vi "CPP-BLplotter.vi"(1 "Job Directory":path) -> (2 "Saved Automatically?":bool, 3 "gnuplotScript":string, 4 "Plot data file":path)   [LabVIEW 2021]
uses:
  gnuplotScriptComponents/BLPlottersubVIs/BLTarget.ctl
  gnuplotScriptComponents/BLPlottersubVIs/Resampler.ctl
  gnuplotScriptComponents/at.ctl
  Results_plotter_Global.vi
  Data plotting/subVIs/Plot_Values_Global.vi
panel:
  in  "Tab Control":enum32{"Good Shit", "Targets", "Boring Shit"}(tab)
  in  "chooseSpectra":bool
  in  "Ref":enum32{"MS", "FS"}(radio)
  in  "Zref":dbl=508.0 min=0.0 step=25.0
  in  "h":dbl[unit] min=0.0 step=0.0005
  in  "NormaliseHeight?":bool
  in  "oneshot":bool=TRUE
  in  "U(h)":dbl[unit] min=0.0 step=0.5
  in  "Fit Zmin(mm)":dbl=100.0 min=0.0 max=200.0 step=20.0
  in  "autoprint":bool
  out "Power fit with d0":cluster{"n":dbl, "d0":dbl, "d0 2":dbl} {"d0 2" format="%#.1e"; "d0" format="%#.1f"; "n" format="%.3f"}
  in  "Fit Zmax(mm)":dbl=550.0 min=0.0 max=2000.0 step=50.0
  out "lambda-":dbl format="%_2g"
  out "lambda+":dbl format="%_2g"
  out "lambda(h)":dbl format="%.3g"
  in  "HeightJitter%":dbl min=0.0 max=20.0 step=1.0
  out "Spectrum":cluster{"all rows":dbl[], "all rows":dbl[]}[](graph)
  in  "Stop Button":bool
  in  "Print Button":bool
  out "U,L(U)":cluster{"Array":dbl[], "Array":dbl[]}[](graph)
  out "TI,Sigma":cluster{"Array":dbl[], "Array":dbl[]}[](graph)
  in  "MaxFitFreq":dbl=500.0
  in  "lambdaSpan(%)":dbl=20.0
  out "case":string
  out "Power fit No d0":cluster{"n":dbl, "d0":dbl, "d0 2":dbl} {"d0 2" format="%#.1e"; "n" format="%.3f"}
  in  "Spectra?":bool
  in  "Scale":u16=350 min=1 max=10000 step=50
  in  "Load BL Targets":bool
  in  "BL Scratchpad":T1[](array[typedef]) {"n" min=0.02 max=0.5 step=0.01 format="%.2f"}
  out "BL Targets":T1[](array[typedef]) {"n" min=0.02 max=0.5 step=0.01 format="%.2f"}
  out "FileName":string
  in  "Values to include in Page Title":i32[](listbox)
  out "ZrefMSmm":dbl
  in  "Units":enum16{"Metric", "English"}(ring)
  out "filenameNotes":string
  in  "ScaleInTitle?":bool
  in  "OutputType":enum16{"PDF", "PNG-ReportStyle"}(ring)
  out "outputPath":path
  in  "Resampler":T2
  in  "ResampleToN":i32=12
  in  "ResampleHeights":dbl[](array[numeric])=[25.4, 38.1, 50.8, 76.2, 101.6, 127.0, 152.4, 203.2, 254.0, 304.8, 406.4, 508.0, 609.6, 812.8, 1219.2, 1524.0]
  in  "Use for:":T3(array[ring])=[enum."\nU", enum."\nTI", enum."\nLambda", enum."\nSigma"]
  out "Incoming Titles":string[](array[string])
  out "Final Title":string
  in  "Plot Title Post Block":string
  in  "Plot Title Pre Block":string="Test"
  in  "Show Script Editor?":bool
  in  "OpenLogfile?":bool
  out "spectraLegend":string[](array[string])
  in  "SpecificPlotFolder":string="EnterSpecificPlotFolder"
  # "Fit using values at  measurement Z heights"
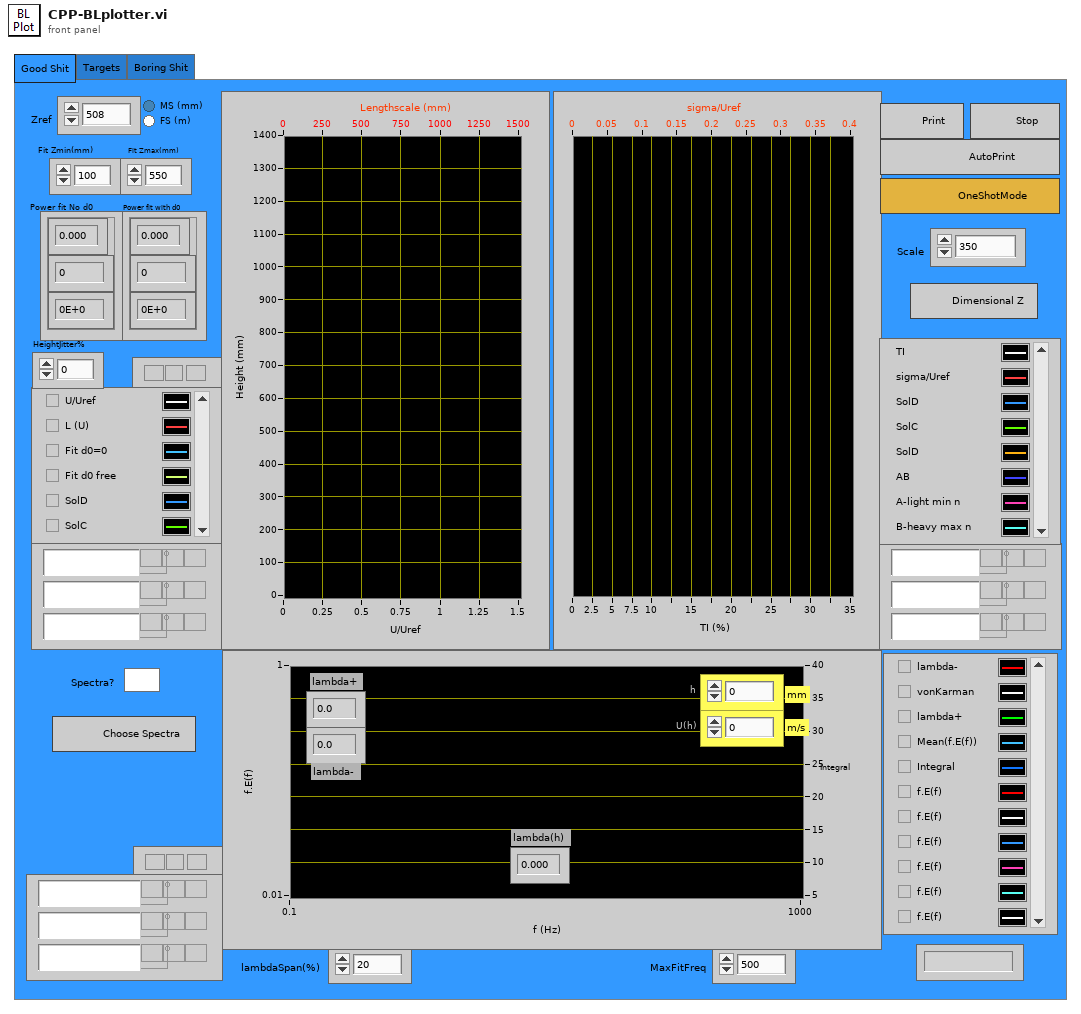
[diagram p1: front panel]
types:
  T1 = typedef "BLTarget.ctl" = cluster{"Code":string, "n":dbl, "Z:FS:(m)":dbl[], "U:FS:(m/s)":dbl[], "TI::(%)":dbl[]}
  T2 = typedef "Resampler.ctl" = enum32{"AsTaken", "Regular", "Prescribed"}
  T3 = enum16{"Don't Use", "\nU", "\nLambda", "\nTI", "\nSigma"}[]
  T4 = typedef "Error_bars.ctl" = cluster{"Upper":string[], "Lower":string[], "St Error":string[]}
  T5 = typedef "at.ctl" = cluster{"XcoordSys":string, "YcoordSys":string, "Xvalue":dbl, "Yvalue":dbl}
  T6 = typedef "LVRangeTypeDef.ctl" = cluster{"Minimum":dbl, "Maximum":dbl, "Increment":dbl, "Minor Increment":dbl, "Start":dbl}
  T7 = typedef "PowerLaw.ctl" = cluster{"n":dbl, "d0":dbl, "Residual":dbl}
  T8 = cluster{"Array":dbl[], "best nonlinear fit":dbl[]}
  T9 = cluster{"Plot.Plot Name":string, "Plot.Plot Color":u32, "Plot.Visible?":bool}
  T10 = typedef "minAndMax.ctl" = cluster{"Min":T11, "Max":T11}
  T11 = typedef "AutoManualNumber.ctl" = cluster{"Auto":bool, "Value":dbl}
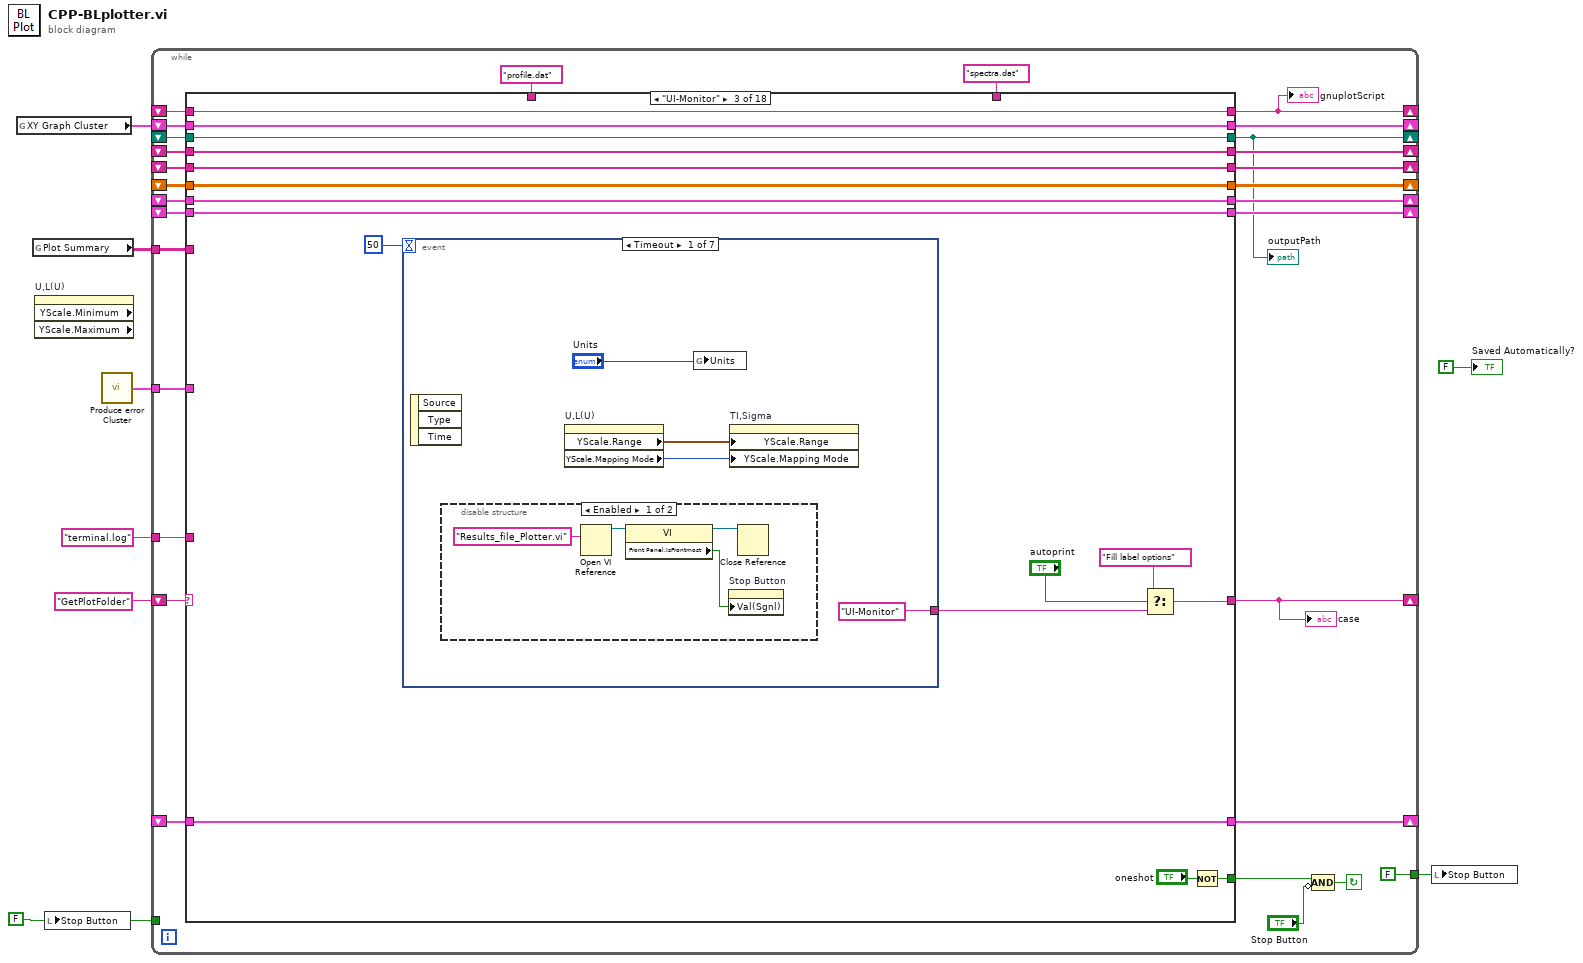
[diagram p0: block diagram]
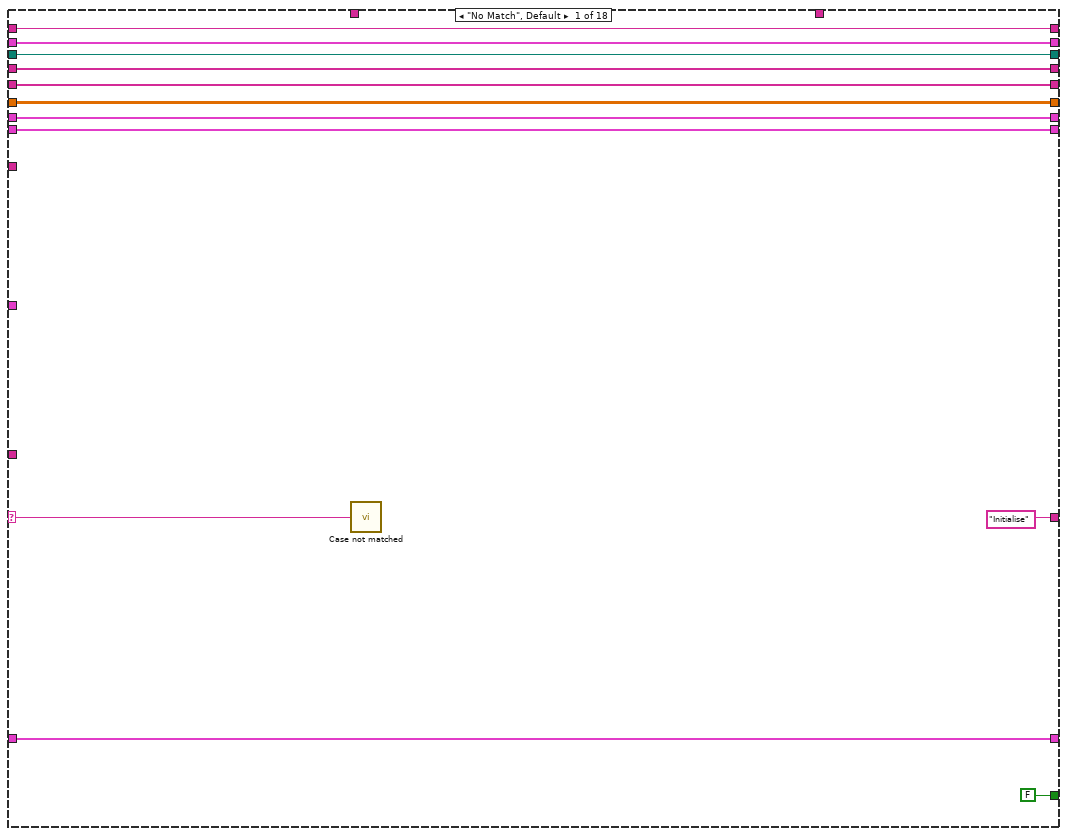
[diagram p2: hidden frame]
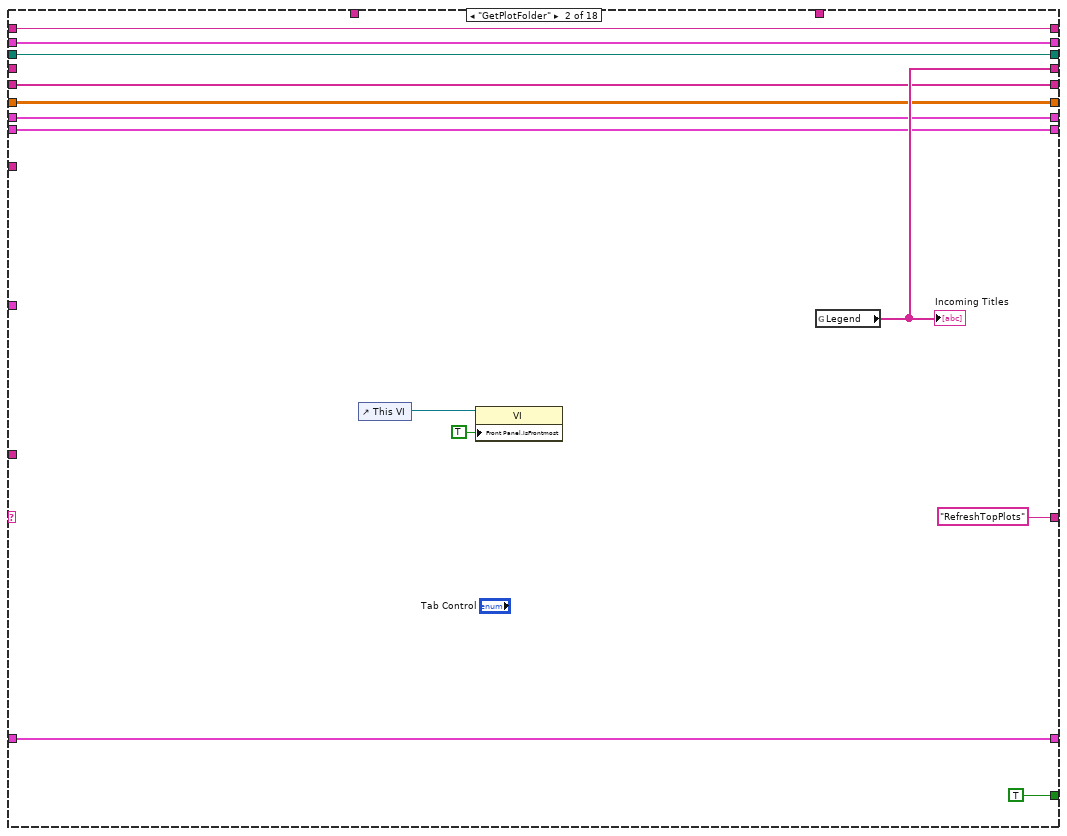
[diagram p3: hidden frame]
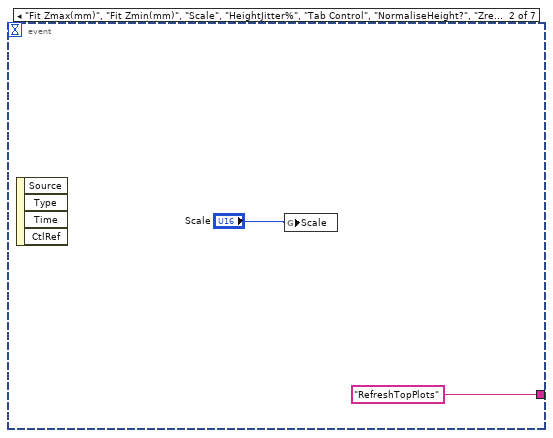
[diagram p5: hidden frame]
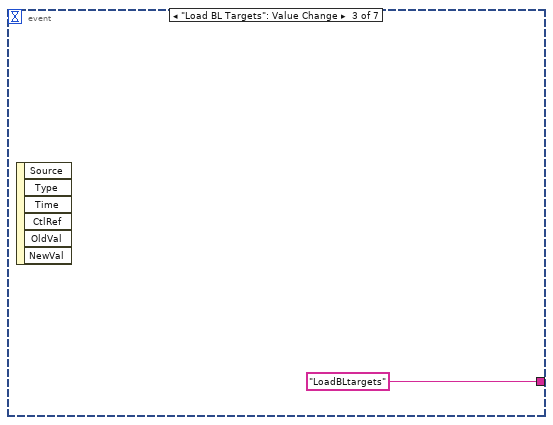
[diagram p6: hidden frame]
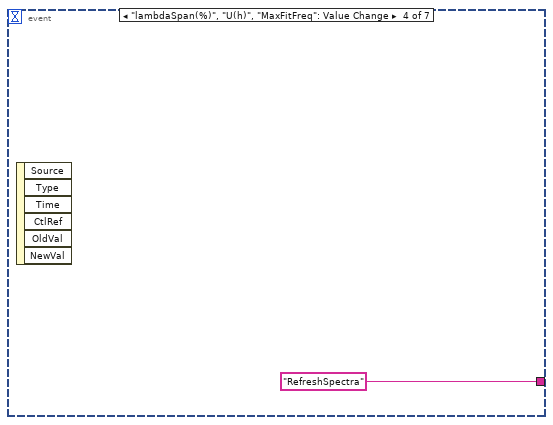
[diagram p7: hidden frame]
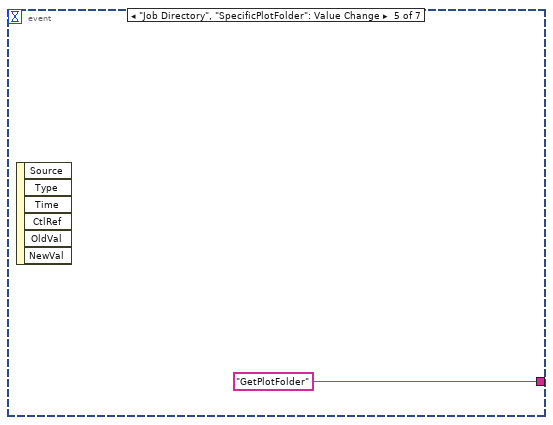
[diagram p8: hidden frame]
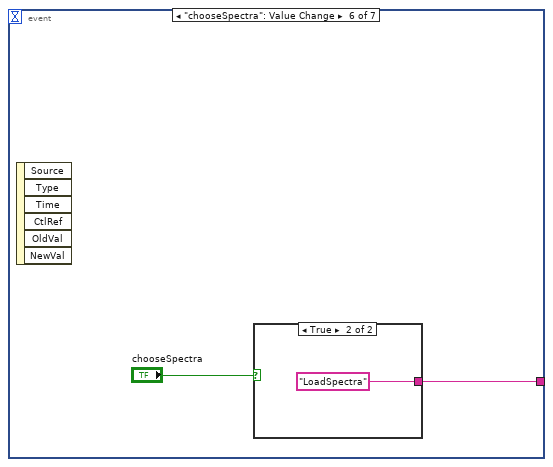
[diagram p9: hidden frame]
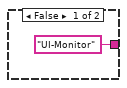
[diagram p10: hidden frame]
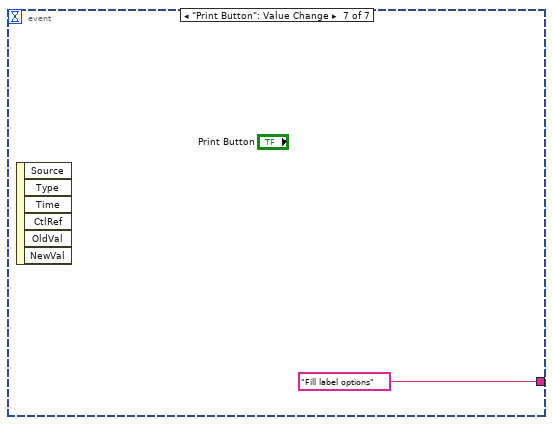
[diagram p11: hidden frame]
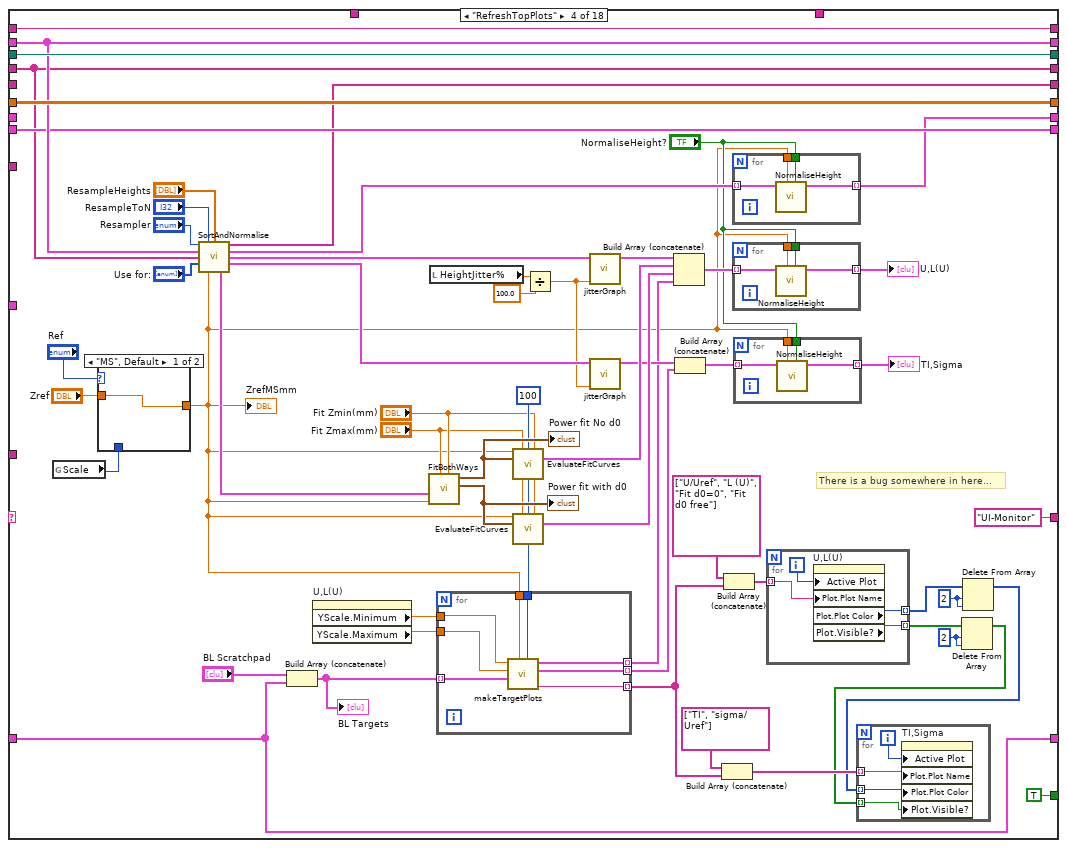
[diagram p12: hidden frame]
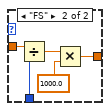
[diagram p13: hidden frame]
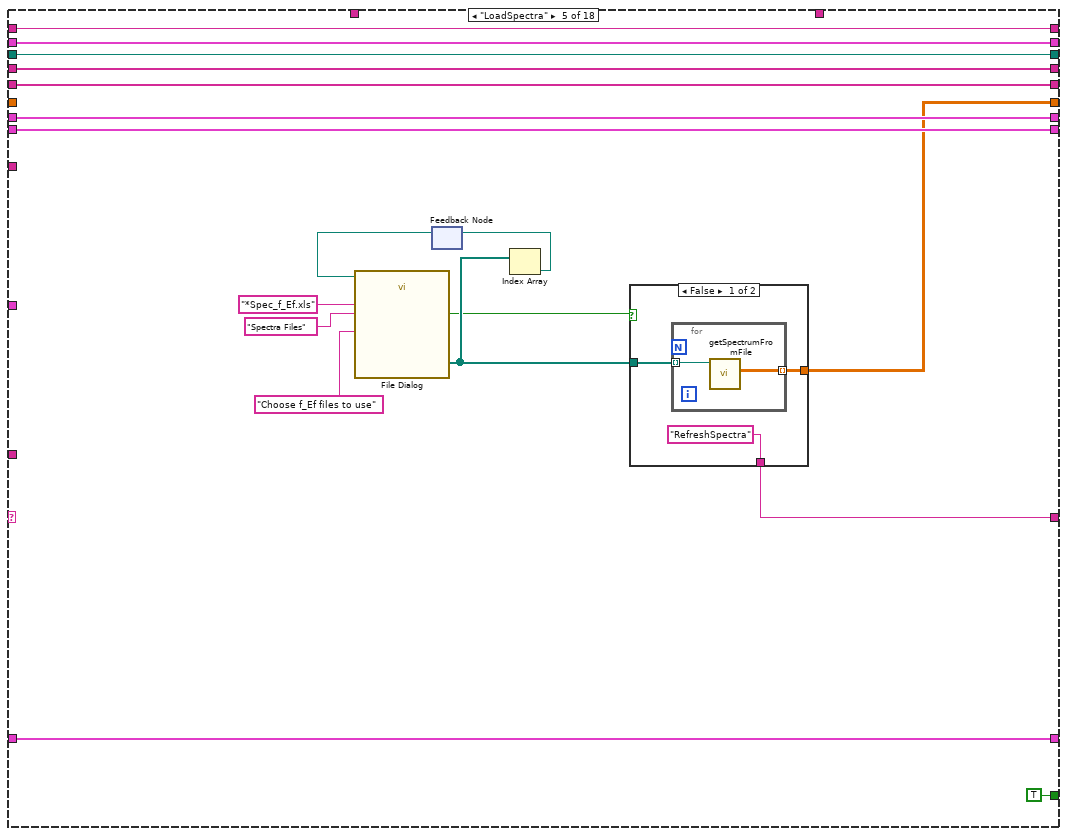
[diagram p14: hidden frame]
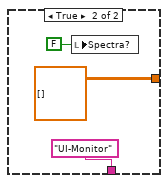
[diagram p15: hidden frame]
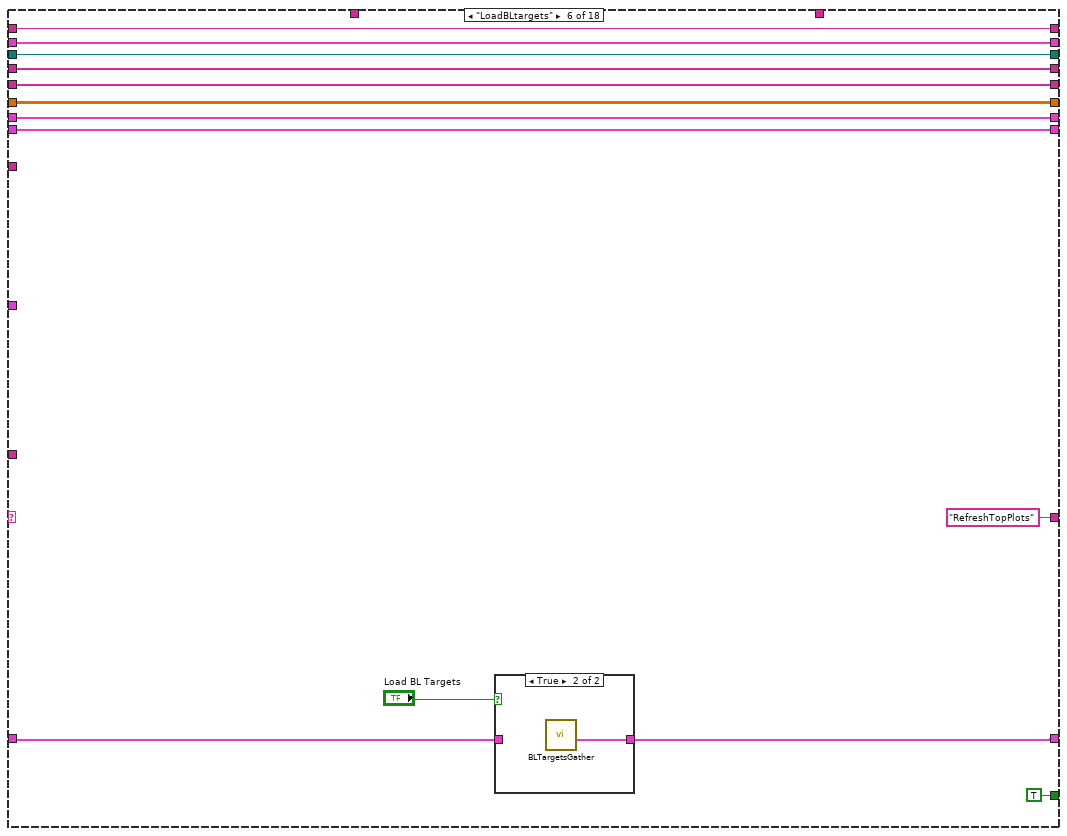
[diagram p16: hidden frame]
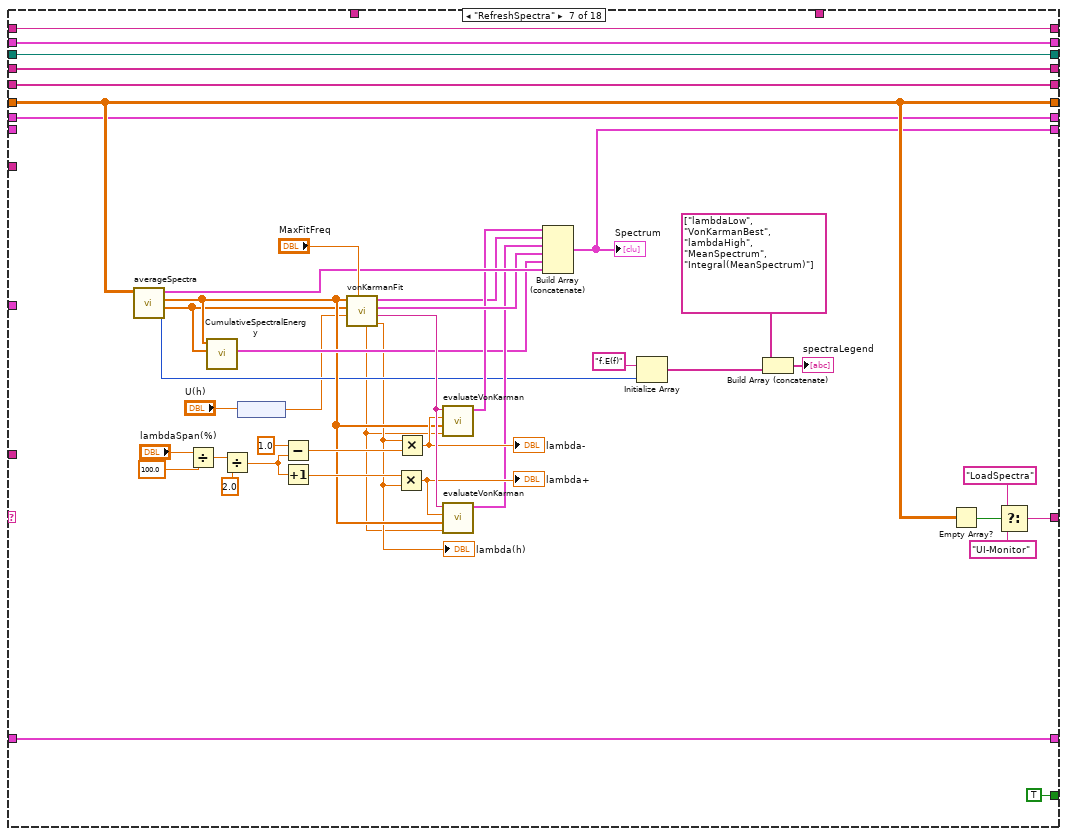
[diagram p18: hidden frame]
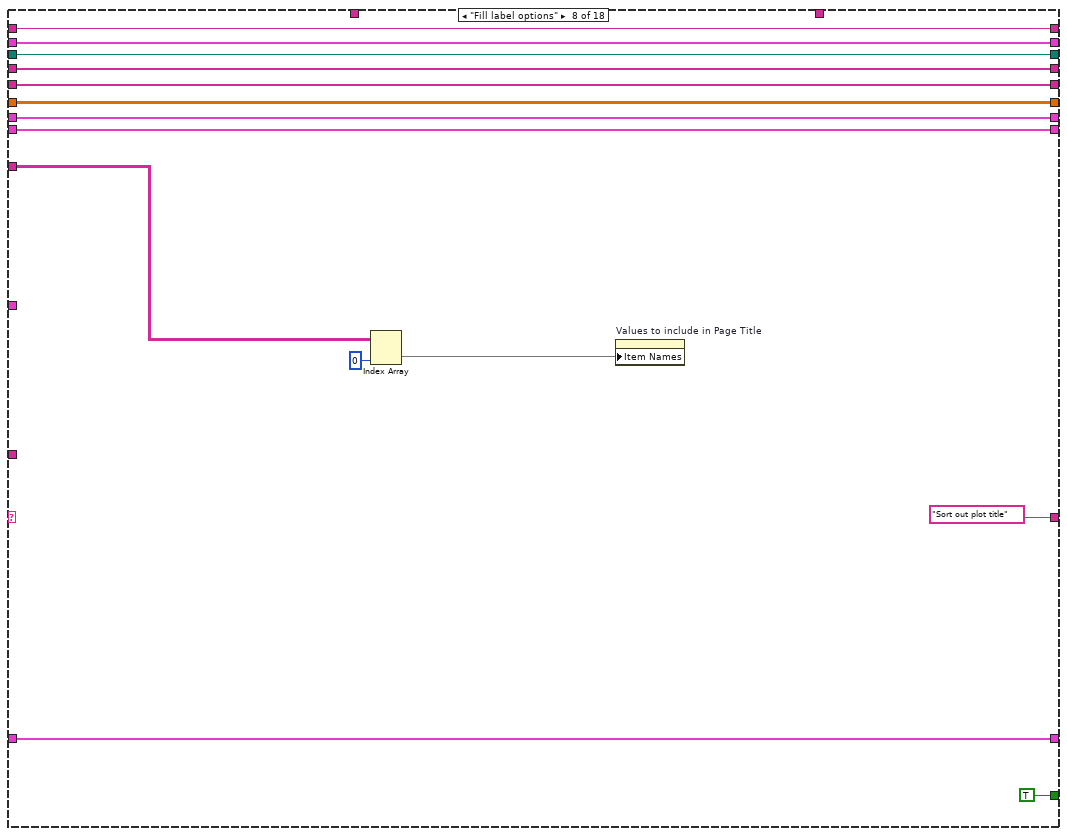
[diagram p19: hidden frame]
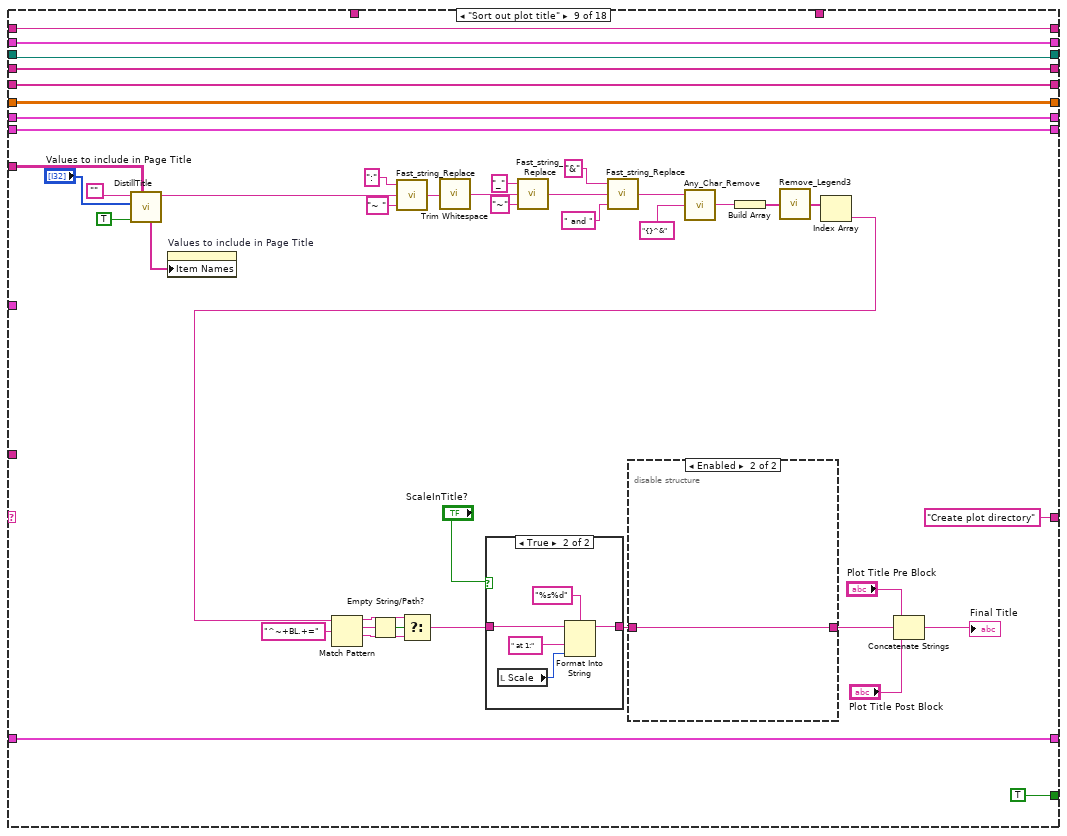
[diagram p20: hidden frame]
diagram:
  w1 = FALSE
  n1 = global read "Plot_Values_Global.vi" "XY Graph Cluster"() -> (w3:cluster{dbl[], dbl[]}[])
  n2 = global read "Results_plotter_Global.vi" "Plot Summary"() -> (w7:string[][])
  n3 = property on="U,L(U)" class="XYGraph (strict)" props=["YScale", "Minimum", "YScale", "Maximum"]() -> ()  [unwired: 2 in, 4 out]
  n4 = local write "Stop Button"(w1) -> ()
  n5 = call "Produce error Cluster.vi"() -> ("Error Bar Cluster"=w4:T4[])  [unwired: 1 in]
  n6 = while {
    shift-left: "GetPlotFolder" -> [w37]
    shift-right: [w30] -> _
    tunnel: w7 -> [w36]
    shift-right: [w15] -> _
    shift-left: _ -> [w35]
    shift-right: [w21] -> _
    shift-left: w3 -> [w34]
    shift-right: [w27] -> _
    shift-left: _ -> [w33]
    shift-right: [w19] -> _
    shift-left: _ -> [w32]
    tunnel: "terminal.log" -> [w31]
    shift-right: [w29] -> _
    shift-left: _ -> [w28]
    shift-right: [w26] -> _
    shift-left: _ -> [w25]
    shift-right: [w22] -> _
    shift-left: _ -> [w20]
    shift-right: [w18] -> _
    shift-left: _ -> [w17]
    tunnel: w4 -> [w16]
    shift-right: [w13] -> _
    shift-left: _ -> [w14]
    tunnel: [FALSE ("Stop Button")] -> w2
    tunnel: w1 -> [_]
    stop <- w9 continue-if-true
    n7 = case shown="\"UI-Monitor\"" w37 {
      selector: w37 -> [w38 _ _ _ _ _ _ _ _ _ _ _ _ _ _ _ _ _]
      tunnel: [FALSE TRUE w63 TRUE ("Top Level") TRUE ("Top Level") TRUE ("Top Level") TRUE ("Top Level") TRUE ("Top Level") TRUE ("Top Level") TRUE TRUE ("Top Level") TRUE ("Top Level") TRUE ("Top Level") TRUE ("Top Level") TRUE ("Top Level") w602 TRUE ("Top Level") TRUE ("Top Level")] -> w10
      tunnel: ["Initialise" "RefreshTopPlots" w69 "UI-Monitor" ("t") w195 "RefreshTopPlots" ("t") w246 "Sort out plot title" "Create plot directory" ("t") "Save .dat file" "Gnuplot script Start" w436 "Write gnuplot file" ("t") "Execute shell script" ("t") "Has pdf been generated?" ("t") w611 "UI-Monitor" ("t") "UI-Monitor" ("t")] -> w30
      tunnel: w36 -> [_ _ _ _ _ _ _ w285 w316 _ w396 _ _ _ _ _ _ _]
      tunnel: [w47 w53 w75 w153 w205 w226 w271 w280 w323 w351 w388 w441 w525 w566 w578 w614 w623 w633] -> w15
      tunnel: w35 -> [w47 w53 w75 w153 w205 w226 w271 w280 w323 _ w388 w441 w525 w566 w578 w614 w623 w633]
      tunnel: w34 -> [w46 w59 w76 w147 w204 w225 w270 w281 w329 w380 w398 w446 w524 w576 w591 w617 w629 w643]
      tunnel: [w46 w59 w76 w147 w204 w225 w270 w281 w329 w380 w398 w446 w524 w576 w591 w617 w629 w643] -> w21
      tunnel: w33 -> [w45 w60 w77 w152 w203 w224 w269 w282 w327 w379 w402 _ w510 w561 w589 w615 w627 w641]
      tunnel: [w45 w60 w77 w152 w203 w224 w269 w282 w327 w379 w402 w419 w514 w561 w589 w615 w627 w641] -> w27
      tunnel: [w44 w58 w74 w138 w202 w223 w268 w279 w328 w378 w399 w445 w523 w571 w590 w616 w628 w642] -> w19
      tunnel: w32 -> [w44 _ w74 w138 w202 w223 w268 w279 w328 w378 w399 w445 w523 w571 w590 w616 w628 w642]
      tunnel: w31 -> [_ _ _ _ _ _ _ _ _ _ _ _ _ _ w586 _ _ w637]
      tunnel: [w43 w57 w78 w151 w196 w217 w241 w278 w325 w375 w397 w443 w522 w568 w585 w607 w625 w635] -> w29
      tunnel: w28 -> [w43 w57 w78 w151 _ w217 w241 w278 w325 w375 w397 w443 w522 w568 w585 w607 w625 w635]
      tunnel: [w42 w56 w72 w140 w200 w220 w240 w277 w324 w374 w392 w442 w521 w567 w584 w606 w624 w634] -> w26
      tunnel: w25 -> [w42 w56 w72 w140 w200 w220 _ w277 w324 w374 w392 w442 w521 w567 w584 w606 w624 w634]
      tunnel: "profile.dat" ("name or relative path") -> [_ _ _ _ _ _ _ _ _ _ w395 w429 _ _ _ _ _ _]
      tunnel: "spectra.dat" ("name or relative path") -> [_ _ _ _ _ _ _ _ _ _ w394 _ w513 _ _ _ _ _]
      tunnel: [w41 w55 w71 w106 w199 w219 w234 w275 w321 w373 w390 w440 w520 w565 w583 w605 w622 w632] -> w22
      tunnel: w20 -> [w41 w55 w71 _ w199 w219 w234 w275 w321 w373 w390 w440 w520 w565 w583 w605 w622 w632]
      tunnel: [w40 w54 w70 w137 w198 w218 w233 w274 w320 w372 w391 w439 w519 w564 w582 w604 w621 w631] -> w18
      tunnel: w17 -> [w40 w54 w70 _ w198 w218 w233 w274 w320 w372 w391 w439 w519 w564 w582 w604 w621 w631]
      tunnel: w16 -> [_ _ _ _ _ _ _ _ _ _ w385 _ _ _ _ _ _ _]
      tunnel: w14 -> [w39 w52 w65 w113 w197 w214 w232 w273 w319 w366 w383 w430 w498 w559 w581 w600 w619 w630]
      tunnel: [w39 w52 w65 w113 w197 w216 w232 w273 w319 w366 w383 w430 w498 w559 w581 w600 w619 w630] -> w13
      frame "No Match", Default {
        n8 = call "Case not matched.vi"("Case Name not Matched"=w38) -> ()
      }
      frame "GetPlotFolder" {
        n9 = control-ref of="This VI"() -> (w50:refnum<vi>)
        n10 = property class="VI"(reference=w50, "Front Panel.IsFrontmost"=TRUE ("Front Panel Window:Is Frontmost")) -> ()  [unwired: 1 in, 2 out]
        n11 = global read "Results_plotter_Global.vi" "Legend"() -> (w58:string[])
        "Incoming Titles" <- w58
      }
      frame "UI-Monitor" {
        n12 = event shown="[0] Timeout" {
          selector: _ -> [_ _ _ _ _ _ _]
          dyn-events: _ -> [_ _ _ _ _ _ _]
          timeout: 50 -> [_ _ _ _ _ _ _]
          tunnel: ["UI-Monitor" "RefreshTopPlots" "LoadBLtargets" "RefreshSpectra" "GetPlotFolder" w93 "Fill label options"] -> w66
          event Timeout {
            n13 = event-data() -> ()  [unwired: 1 in, 3 out]
            n14 = disable-structure shown="Enabled" {
              frame Enabled {
                n15 = Open VI Reference(vi path="Results_file_Plotter.vi") -> (vi reference=w85:refnum<vi>)  [unwired: 5 in, 1 out]
                n16 = property class="VI"(reference=w85) -> (reference out=w86:refnum<vi>, "Front Panel.IsFrontmost"=w84:bool)  [unwired: 1 in, 1 out]
                n17 = property on="Stop Button" class="Bool (strict)"("Val(Sgnl)"=w84) -> ()  [unwired: 2 in, 2 out]
                n18 = Close Reference(reference=w86) -> ()  [unwired: 1 in, 1 out]
              }
              frame Disabled {
              }
            }
            n19 = property on="U,L(U)" class="XYGraph (strict)"() -> ("YScale.Range"=w80:T6, "YScale.Mapping Mode"=w81:u8)  [unwired: 2 in, 2 out]
            n20 = global write "Results_plotter_Global.vi" "Units"("Units") -> ()
            n21 = property on="TI,Sigma" class="XYGraph (strict)"("YScale.Range"=w80, "YScale.Mapping Mode"=w81) -> ()  [unwired: 2 in, 2 out]
          }
          event "Fit Zmax(mm)", "Fit Zmin(mm)", "Scale", "HeightJitter%", "Tab Control", "NormaliseHeight?", "Zref", "Ref": Value Change; "U,L(U)": Plot Attribute Change {
            n22 = event-data() -> ()  [unwired: 1 in, 4 out]
            n23 = global write "Results_plotter_Global.vi" "Scale"("Scale") -> ()
          }
          event "Load BL Targets": Value Change {
            n24 = event-data() -> ()  [unwired: 1 in, 6 out]
          }
          event "lambdaSpan(%)", "U(h)", "MaxFitFreq": Value Change {
            n25 = event-data() -> ()  [unwired: 1 in, 6 out]
          }
          event "Job Directory", "SpecificPlotFolder": Value Change {
            n26 = event-data() -> ()  [unwired: 1 in, 6 out]
          }
          event "chooseSpectra": Value Change {
            n27 = event-data() -> ()  [unwired: 1 in, 6 out]
            n28 = case shown="True" "chooseSpectra" {
              tunnel: ["UI-Monitor" "LoadSpectra"] -> w93
              frame False {
              }
              frame True {
              }
            }
          }
          event "Print Button": Value Change {
            n29 = event-data() -> ()  [unwired: 1 in, 6 out]
          }
        }
        n30 = Select(t="Fill label options", s="autoprint", f=w66) -> (s? t:f=w69:string)
        n31 = Not(x="oneshot") -> (.not. x?=w63:bool)
      }
      frame "RefreshTopPlots" {
        w121 = 2 ("length")
        w122 = 2 ("length")
        w105 = 100
        # "There is a bug somewhere in here..."
        n32 = global read "Results_plotter_Global.vi" "Scale"() -> (w98:u16)
        n33 = case shown="\"MS\", Default" "Ref" {
          tunnel: "Zref" -> [w154 w157]
          tunnel: w98 -> [_ w156]
          tunnel: [w154 w155] -> w97
          frame "MS", Default {
          }
          frame "FS" {
            n34 = Divide(x=w157, y=w156) -> (x/y=w159:dbl)
            n35 = Multiply(x=w159, y=1000.0) -> (x*y=w155:dbl)
          }
        }
        "ZrefMSmm" <- w97
        n36 = call "SortAndNormalise.vi"("Resampler"="Resampler", "ResampleToN"="ResampleToN", "ResampleHeights"="ResampleHeights", "Plot Array In"=w147, "LegendsIn"=w138, "Use for:"="Use for:", "Zref"=w97) -> ("SortedLegends"=w137:string[], "SortedData"=w107:cluster{"Array":dbl[], "Array":dbl[]}[], "LeftGraph"=w144:cluster{"Array":dbl[], "Array":dbl[]}[], "RightGraph"=w142:cluster{"Array":dbl[], "Array":dbl[]}[], "UzClusterOutput"=w112:cluster{"Array":dbl[], "Array":dbl[]})  [unwired: 4 in]
        n37 = Build Array (concatenate)("BL Scratchpad", w113) -> (w118:T1[])
        "BL Targets" <- w118
        n38 = property on="U,L(U)" class="XYGraph (strict)"() -> ("YScale.Minimum"=w135:dbl, "YScale.Maximum"=w134:dbl)  [unwired: 2 in, 2 out]
        n39 = call "FitBothWays.vi"("Fit Zmin"="Fit Zmin(mm)", "Fit Zmax"="Fit Zmax(mm)", "Zref"=w97, "zUCluster in"=w112) -> ("PowerLawWithDisplacement"=w132:T7, "PowerLawNoDisplacement"=w133:T7)  [unwired: 6 in]
        "Power fit No d0" <- w133
        "Power fit with d0" <- w132
        n40 = local read "HeightJitter%"() -> (w149:dbl)
        n41 = for {
          tunnel: w105 -> [w184]
          tunnel: w135 -> [w181]
          tunnel: w134 -> [w180]
          tunnel: w118 -> [w187] mode=indexing
          tunnel: [w183] -> w129 mode=indexing
          tunnel: [w182] -> w128 mode=indexing
          tunnel: w97 -> [w185]
          tunnel: [w186] -> w101 mode=indexing
          n42 = call "makeTargetPlots.vi"("nPoints"=w184, "ZrefMSmm"=w185, "Cluster"=w187, "Fit Zmax"=w180, "Fit Zmin"=w181) -> ("Code"=w182:string, "TIzClusterOut"=w183:cluster{"TI::(%)":dbl[], "Array":dbl[]}, "UzClusterOutput"=w186:cluster{dbl[], dbl[]})  [unwired: 4 in]
        }
        n43 = call "EvaluateFitCurves.vi"("Zref"=w97, "Fit Zmax"="Fit Zmax(mm)", "nPoints"=w105, "Fit Zmin"="Fit Zmin(mm)", "PowerLaw"=w133) -> ("PlotCluster"=w139:cluster{"Array":dbl[], "Array":dbl[]})  [unwired: 10 in]
        n44 = call "EvaluateFitCurves.vi"("Zref"=w97, "Fit Zmax"="Fit Zmax(mm)", "nPoints"=w105, "Fit Zmin"="Fit Zmin(mm)", "PowerLaw"=w132) -> ("PlotCluster"=w136:cluster{"Array":dbl[], "Array":dbl[]})  [unwired: 10 in]
        n45 = Divide(x=w149, y=100.0) -> (x/y=w141:dbl)
        n46 = call "jitterGraph.vi"("Y-jitter"=w141, "GraphPlots"=w144) -> ("jitteredGraphPlots"=w143:cluster{"Array":dbl[], "Array":dbl[]}[])  [unwired: 9 in]
        n47 = call "jitterGraph.vi"("Y-jitter"=w141, "GraphPlots"=w142) -> ("jitteredGraphPlots"=w130:cluster{"Array":dbl[], "Array":dbl[]}[])  [unwired: 9 in]
        n48 = Build Array (concatenate)(w143, w139, w136, w101) -> (w111:cluster{"Array":dbl[], "Array":dbl[]}[])
        n49 = Build Array (concatenate)(w130, w129) -> (w109:cluster{"TI::(%)":dbl[], "Array":dbl[]}[])
        n50 = Build Array (concatenate)(string[] ["TI", "sigma/Uref"], w128) -> (w131:string[])
        n51 = Build Array (concatenate)(string[] ["U/Uref", "L (U)", "Fit d0=0", "Fit d0 free"], w128) -> (w125:string[])
        n52 = for {
          tunnel: w107 -> [w163] mode=indexing
          tunnel: [w162] -> w106 mode=indexing
          tunnel: w97 -> [w161]
          tunnel: "NormaliseHeight?" -> [w160]
          n53 = call "NormaliseHeight.vi"("NormaliseHeight?"=w160, "Zref"=w161, "Value-Z Cluster In"=w163) -> ("Value-Z Cluster Out"=w162:cluster{"Array":dbl[], "Array":dbl[]})  [unwired: 8 in]
        }
        n54 = for {
          tunnel: w111 -> [w171] mode=indexing
          tunnel: [w170] -> w110 mode=indexing
          tunnel: w97 -> [w169]
          tunnel: "NormaliseHeight?" -> [w168]
          n55 = call "NormaliseHeight.vi"("NormaliseHeight?"=w168, "Zref"=w169, "Value-Z Cluster In"=w171) -> ("Value-Z Cluster Out"=w170:cluster{"Array":dbl[], "Array":dbl[]})  [unwired: 8 in]
        }
        "U,L(U)" <- w110
        n56 = for {
          tunnel: w109 -> [w167] mode=indexing
          tunnel: [w166] -> w108 mode=indexing
          tunnel: w97 -> [w165]
          tunnel: "NormaliseHeight?" -> [w164]
          n57 = call "NormaliseHeight.vi"("NormaliseHeight?"=w164, "Zref"=w165, "Value-Z Cluster In"=w167) -> ("Value-Z Cluster Out"=w166:cluster{"Array":dbl[], "Array":dbl[]})  [unwired: 8 in]
        }
        "TI,Sigma" <- w108
        n58 = for {
          tunnel: w125 -> [w176] mode=indexing
          tunnel: [w179] -> w124 mode=indexing
          tunnel: [w178] -> w120 mode=indexing
          i -> [w177]
          n59 = property on="U,L(U)" class="XYGraph (strict)"("Active Plot"=w177, "Plot.Plot Name"=w176) -> ("Plot.Plot Color"=w179:u32, "Plot.Visible?"=w178:bool)  [unwired: 2 in, 2 out]
        }
        n60 = Delete From Array(array=w120, length=w121, index=w121) -> (array with subset deleted=w119:bool[])  [unwired: 1 out]
        n61 = Delete From Array(array=w124, length=w122, index=w122) -> (array with subset deleted=w123:u32[])  [unwired: 1 out]
        n62 = for {
          tunnel: w131 -> [w172] mode=indexing
          tunnel: w123 -> [w175] mode=indexing
          tunnel: w119 -> [w174] mode=indexing
          i -> [w173]
          n63 = property on="TI,Sigma" class="XYGraph (strict)"("Active Plot"=w173, "Plot.Plot Name"=w172, "Plot.Plot Color"=w175, "Plot.Visible?"=w174) -> ()  [unwired: 2 in, 2 out]
        }
      }
      frame "LoadSpectra" {
        n64 = feedback #1() -> (w189:path)  [unwired: 1 in]
        n65 = call "File Dialog"("start path"=w189, "prompt"="Choose f_Ef files to use", "pattern (all files)"="*Spec_f_Ef.xls" ("pattern"), "pattern label"="Spectra Files") -> ("selected paths"=w191:path[], "cancelled"=w188:bool)  [unwired: 8 in, 2 out]
        n66 = Index Array(array=w191) -> (element=w190:path)  [unwired: 1 in]
        n67 = feedback-in #1(w190) -> ()
        n68 = case shown="False" w188 {
          tunnel: [w208 dbl[][][] [] ("array")] -> w196
          tunnel: w191 -> [w207 _]
          tunnel: ["RefreshSpectra" ("t") "UI-Monitor" ("t")] -> w195
          frame False {
            n69 = for {
              tunnel: w207 -> [w209] mode=indexing
              tunnel: [w210] -> w208 mode=indexing
              n70 = call "getSpectrumFromFile.vi"("File Path Control"=w209) -> ("array"=w210:dbl[][])  [unwired: 10 in]
            }
          }
          frame True {
            n71 = local write "Spectra?"(FALSE ("Spectra?")) -> ()
          }
        }
      }
      frame "LoadBLtargets" {
        n72 = case shown="True" "Load BL Targets" {
          tunnel: [w227 w228] -> w216
          tunnel: w214 -> [w227 _]
          frame False {
          }
          frame True {
            n73 = call "BLTargetsGather.vi"() -> ("BL Targets out"=w228:T1[])  [unwired: 11 in]
          }
        }
      }
      frame "RefreshSpectra" {
        n74 = call "averageSpectra.vi"("multipleSpectra"=w241) -> ("nSpectra"=w238:i32, "meanSpectrum"=w242:dbl[], "frequencies"=w243:dbl[], "spectraPlots"=w265:cluster{"Array":dbl[], "Array":dbl[]}[])  [unwired: 7 in]
        n75 = Divide(x="lambdaSpan(%)", y=100.0) -> (x/y=w258:dbl)
        n76 = call "CumulativeSpectralEnergy.vi"("f.E(f)"=w242, "f"=w243) -> ("plottableBundle"=w249:cluster{"X":dbl[], "Array":dbl[]})  [unwired: 8 in, 1 out]
        n77 = Divide(x=w258, y=2.0 ("x")) -> (x/y=w251:dbl)
        n78 = node("U(h)") -> (w229:dbl)
        n79 = Subtract(x=1.0, y=w251) -> (x-y=w260:dbl)
        n80 = Increment(x=w251) -> (x+1=w259:dbl)
        n81 = call "vonKarmanFit.vi"("MaxFitFreq"="MaxFitFreq", "U(h)"=w229, "f.E(f)"=w242, "f"=w243) -> ("lambda"=w231:dbl, "vonKarmanFitEquation"=w263:string, "CroppedData"=w264:cluster{"X Out":dbl[], "Y Out":dbl[]}, "FitCurve"=w253:T8, "a"=w230:dbl)  [unwired: 3 in]
        "lambda(h)" <- w231
        n82 = Multiply(x=w259, y=w231) -> (x*y=w254:dbl)
        "lambda+" <- w254
        n83 = Multiply(x=w231, y=w260) -> (x*y=w255:dbl)
        "lambda-" <- w255
        n84 = call "evaluateVonKarman.vi"("a"=w230, "frequencies"=w243, "lambda"=w255, "vonKarmanFitEquation"=w263) -> ("Cluster"=w256:cluster{"frequencies":dbl[], "Y Values":dbl[]})  [unwired: 7 in]
        n85 = call "evaluateVonKarman.vi"("a"=w230, "frequencies"=w243, "lambda"=w254, "vonKarmanFitEquation"=w263) -> ("Cluster"=w252:cluster{"frequencies":dbl[], "Y Values":dbl[]})  [unwired: 7 in]
        n86 = Build Array (concatenate)(w256, w253, w252, w264, w249, w265) -> (w240:cluster{"Array":dbl[], "Array":dbl[]}[])
        "Spectrum" <- w240
        n87 = Initialize Array("f.E(f)", w238) -> (w237:string[])
        n88 = Build Array (concatenate)(string[] ["lambdaLow", "VonKarmanBest", "lambdaHigh", "MeanSpectrum", "Integral(MeanSpectrum)"], w237) -> (→"spectraLegend":string[])
        n89 = Empty Array?(array=w241) -> (empty?=w245:bool)
        n90 = Select(t="LoadSpectra", s=w245, f="UI-Monitor" ("t")) -> (s? t:f=w246:string)
      }
      frame "Fill label options" {
        n91 = Index Array(array=w285, index (col)=0 ("disabled index (col)")) -> (element=w272:string[])  [unwired: 1 in]
        n92 = property on="Values to include in Page Title" class="LstBox (strict)"("Item Names"=w272) -> ()  [unwired: 2 in, 2 out]
      }
      frame "Sort out plot title" {
        n93 = call "DistillTitle.vi"("Plot Summary in"=w316, "Show Channels with range of Values?"=TRUE, "Indices to include in Page Title"="Values to include in Page Title", "String in"="") -> ("String out"=w293:string, "AvailableVariables"=w313:string[])  [unwired: 6 in]
        n94 = property on="Values to include in Page Title" class="LstBox (strict)"("Item Names"=w313) -> ()  [unwired: 2 in, 2 out]
        n95 = call "Fast_string_Replace.vi"("Replace match with:"="~ ", "Input String"=w293, "regular expression"=":") -> ("Output String"=w303:string)  [unwired: 2 out]
        n96 = call <vilib>:"Trim Whitespace.vi"("string"=w303) -> ("trimmed string"=w304:string)  [unwired: 1 in]
        n97 = call "Fast_string_Replace.vi"("Replace match with:"="~", "Input String"=w304, "regular expression"="_") -> ("Output String"=w298:string)  [unwired: 2 out]
        n98 = call "Fast_string_Replace.vi"("Replace match with:"=" and " ("Individual Characters to Remove"), "Input String"=w298, "regular expression"="&" ("Individual Characters to Remove")) -> ("Output String"=w308:string)  [unwired: 1 in, 1 out]
        n99 = call "Any_Char_Remove.vi"("Individual Characters to Remove"="{}^&", "String in"=w308) -> ("String out"=w307:string)  [unwired: 1 in]
        n100 = Build Array(w307) -> (w305:string[])
        n101 = call "Remove_Legend3.vi"("Ordinate Strings"=w305) -> ("Array"=w306:string[])
        n102 = Index Array(array=w306) -> (element=w291:string)  [unwired: 1 in]
        n103 = Match Pattern(string=w291, regular expression="^~+BL.+=") -> (before substring=w288:string, match substring=w290:string, after substring=w287:string)  [unwired: 1 in, 1 out]
        n104 = Empty String/Path?(string/path=w290) -> (empty?=w289:bool)
        n105 = Select(t=w288, s=w289, f=w287) -> (s? t:f=w286:string)
        n106 = case shown="True" "ScaleInTitle?" {
          tunnel: w286 -> [w340 w345]
          tunnel: [w340 w341] -> w317
          frame False {
          }
          frame True {
            n107 = local read "Scale"() -> (w344:u16)
            n108 = Format Into String(format string="%s%d", initial string=w345, " at 1:" ("string"), w344) -> (resulting string=w341:string)  [unwired: 1 in, 1 out]
          }
        }
        n109 = disable-structure shown="Enabled" {
          disable-tunnel: w317 -> [w332 w339]
          disable-tunnel: [w330 w339] -> w297
          frame Disabled {
            n110 = local read "Spectra?"() -> (w331:bool)
            n111 = case shown="True" w331 {
              tunnel: w332 -> [w333 w338]
              tunnel: [w333 w335] -> w330
              frame False {
              }
              frame True {
                n112 = local read "h"() -> (w334:dbl[unit])
                n113 = Format Into String(format string="%s%{mm}d", initial string=w338, " Z=" ("string"), w334) -> (resulting string=w335:string)  [unwired: 1 in, 1 out]
              }
            }
          }
          frame Enabled {
          }
        }
        n114 = Concatenate Strings("Plot Title Pre Block", w297, "Plot Title Post Block") -> (→"Final Title":string)
      }
      frame "Create plot directory" {
        w353 = "" ("replace string (\"\")")
        n115 = local read "Final Title"() -> (w350:string)
        n116 = Search and Replace String(replace all?=TRUE ("replace all? (F)"), input string=w350, search string=",", replace string="_" ("replace string (\"\")")) -> (result string=w364:string)  [unwired: 4 in, 3 out]
        n117 = Search and Replace String(replace all?=TRUE ("replace all? (F)"), input string=w364, search string=" +", replace string=w353) -> (result string=w355:string)  [unwired: 4 in, 3 out]
        n118 = Build Path(base path="Job Directory", name or relative path="BL_plots") -> (appended path=w367:path)
        n119 = Search and Replace String(replace all?=TRUE ("replace all? (F)"), input string=w355, search string="~+", replace string=w353) -> (result string=w356:string)  [unwired: 4 in, 3 out]
        n120 = Build Path(base path=w367, name or relative path="SpecificPlotFolder") -> (appended path=w370:path)
        n121 = call <vilib>:"Is Name Multiplatform.vi"("filename must be valid on all platforms (F)"=TRUE ("name must work for all platforms (F)"), "filename"=w356) -> ("suggested filename"=w349:string, "problem description"=→"filenameNotes":string)  [unwired: 5 in, 3 out]
        n122 = Build Path(base path=w370, name or relative path=w349) -> (appended path=w352:path)
        n123 = call <vilib>:"Create Directory Recursive.vi"("directory"=w352) -> ("directory copy"=w351:path)  [unwired: 4 in, 2 out]
        n124 = Search and Replace String(replace all?=TRUE ("replace all? (F)"), input string=w349, search string="=") -> (result string=→"FileName":string)  [unwired: 5 in, 3 out]
      }
      frame "Save .dat file" {
        w389 = "Profile Plot" ("X Axis Name")
        n125 = local read "ZrefMSmm"() -> (w382:dbl)
        n126 = local read "BL Targets"() -> (w387:T1[])
        n127 = local read "Scale"() -> (w386:u16)
        n128 = call "saveTargetsFile.vi"("BL Targets"=w387, "Path"=w388, "ZrefMSmm"=w382, "Scale"=w386) -> ()  [unwired: 8 in]
        n129 = Build Path(base path=w388, name or relative path=w395) -> (appended path=w381:path)
        "Plot data file" <- w381
        n130 = call "MakeDataFileForMultiplot.vi"("Legend"=w391, "Path"=w381, "Plot Array"=w390, "Plot Summary"=w396, "Transpose"=TRUE, "Error Bar Cluster"=w385, "X Axis Name"=w389, "Y Axis Name"=w389) -> ()  [unwired: 8 in]
        n131 = local read "Spectra?"() -> (w384:bool)
        n132 = case shown="True" w384 {
          tunnel: w396 -> [_ w411]
          tunnel: w394 -> [_ w410]
          tunnel: w392 -> [_ w409]
          tunnel: w389 -> [_ _]
          tunnel: w388 -> [_ w408]
          tunnel: w385 -> [_ w407]
          frame False {
          }
          frame True {
            n133 = local read "spectraLegend"() -> (w403:string[])
            n134 = Build Path(base path=w408, name or relative path=w410) -> (appended path=w404:path)
            n135 = call "MakeDataFileForMultiplot.vi"("Legend"=w403, "Path"=w404, "Plot Array"=w409, "Plot Summary"=w411, "Error Bar Cluster"=w407, "X Axis Name"="f (Hz)", "Y Axis Name"="f.E(f)") -> ()  [unwired: 9 in]
          }
        }
      }
      frame "Gnuplot script Start" {
        # "Number of \"permanent\" plots"
        # "Number of \"permanent\" plots"
        n136 = local read "BL Targets"() -> (w415:T1[])
        n137 = Array Size(array=w415) -> (size(s)=w431:i32)
        n138 = Add(x=w431, y=4 ("x")) -> (x+y=w434:i32)
        n139 = for {
          N: w434 -> [_]
          tunnel: [w476] -> w414 mode=indexing
          i -> [w475]
          n140 = property on="U,L(U)" class="XYGraph (strict)"("Active Plot"=w475) -> ("Plot.Plot Name"=w479:string, "Plot.Plot Color"=w478:u32, "Plot.Visible?"=w477:bool)  [unwired: 2 in, 2 out]
          n141 = Bundle("Plot.Plot Name"=w479, "Plot.Plot Color"=w478, "Plot.Visible?"=w477) -> (w476:T9)  [unwired: 1 in]
        }
        n142 = global write "Results_plotter_Global.vi" "OutputType"("OutputType") -> ()
        n143 = Add(x=w431, y=2 ("x")) -> (x+y=w432:i32)
        n144 = local read "NormaliseHeight?"() -> (w426:bool)
        n145 = local read "Power fit with d0"() -> (w420:cluster{"n":dbl, "d0":dbl, "d0 2":dbl})
        n146 = local read "Power fit No d0"() -> (w421:cluster{"n":dbl, "d0":dbl, "d0 2":dbl})
        n147 = local read "Fit Zmax(mm)"() -> (w424:dbl)
        n148 = local read "Fit Zmin(mm)"() -> (w423:dbl)
        n149 = for {
          N: w432 -> [_]
          tunnel: [w472] -> w413 mode=indexing
          i -> [w470]
          n150 = property on="TI,Sigma" class="XYGraph (strict)"("Active Plot"=w470) -> ("Plot.Plot Name"=w471:string, "Plot.Plot Color"=w474:u32, "Plot.Visible?"=w473:bool)  [unwired: 2 in, 2 out]
          n151 = Bundle("Plot.Plot Name"=w471, "Plot.Plot Color"=w474, "Plot.Visible?"=w473) -> (w472:T9)  [unwired: 1 in]
        }
        n152 = local read "Final Title"() -> (w428:string)
        n153 = control-ref of="TI,Sigma"() -> (w416:refnum<vi>)
        n154 = control-ref of="U,L(U)"() -> (w417:refnum<vi>)
        n155 = local read "Scale"() -> (w418:u16)
        n156 = local read "Zref"() -> (w425:dbl)
        n157 = case shown="\"PDF\", Default" "OutputType" {
          tunnel: w429 -> [w463 _]
          tunnel: w428 -> [w462 w469]
          tunnel: "Spectra?" -> [w461 w468]
          tunnel: w426 -> [w460 _]
          tunnel: w425 -> [w459 w464]
          tunnel: w424 -> [w458 _]
          tunnel: w423 -> [w457 _]
          tunnel: "HeightJitter%" -> [w456 _]
          tunnel: w421 -> [w455 _]
          tunnel: w420 -> [w454 _]
          tunnel: [w453 w467] -> w419
          tunnel: w418 -> [w452 w466]
          tunnel: w417 -> [w451 _]
          tunnel: w416 -> [w450 _]
          tunnel: w415 -> [w449 w465]
          tunnel: w414 -> [w448 _]
          tunnel: w413 -> [w447 _]
          frame "PDF", Default {
            n158 = call "AssembleBLMultiplotScript-UandTI.vi"("name or relative path"=w463, "Final Title"=w462, "Spectra?"=w461, "NormaliseHeight?"=w460, "Zref"=w459, "Fit Zmax"=w458, "Fit Zmin"=w457, "HeightJitter%"=w456, "Scale"=w452, "BL Targets"=w449, "U,L(U)"=w451, "UtargetsInfo"=w448, "TI,Sigma"=w450, "TItargetsInfo"=w447, "No d0"=w455, "with d0"=w454) -> ("gnuplotOut"=w453:string)  [unwired: 11 in]
          }
          frame "PNG-ReportStyle" {
            n159 = call "AssembleBLMultiplotScript-UandTI-CPPPNG.vi"("Final Title"=w469, "Spectra?"=w468, "Zref"=w464, "Scale"=w466, "BL Targets"=w465) -> ("gnuplotOut"=w467:string)  [unwired: 22 in]
          }
        }
        n160 = Select(t="spectraScript", s="Spectra?", f="Write gnuplot file" ("t")) -> (s? t:f=w436:string)
      }
      frame "spectraScript" {
        w509 = 0.0 ("LateralPosition")
        w515 = 0 ("Active Y Scale")
        n161 = global read "Results_plotter_Global.vi" "OutputType"() -> (w495:enum16{"PDF", "PNG-ReportStyle"})
        n162 = global read "Results_plotter_Global.vi" "Scale"() -> (w483:u16)
        n163 = global read "Results_plotter_Global.vi" "Units"() -> (w487:enum16{"Metric", "English"})
        n164 = Greater?(x=w483, y=u16 10) -> (0:w481:bool)
        n165 = case shown="\"PDF\", Default" w495 {
          tunnel: [w530 1.0 ("Width")] -> w508
          tunnel: [w530 0.35 ("Width")] -> w497
          tunnel: ["'\\color{g}{PSD of longitudinal velocity}'" "'PSD of longitudinal velocity'"] -> w496
          tunnel: ["$h= %.0{mm}f$" ("format string") w535] -> w493
          tunnel: ["$U(h)= %0.2{m/s}f$" ("format string") w534] -> w491
          tunnel: ["$\\\\lambda(h)= %0.2f$" ("format string") w533] -> w489
          tunnel: w487 -> [_ w532]
          tunnel: w481 -> [_ w531]
          frame "PDF", Default {
            w530 = 1.0 ("Width")
          }
          frame "PNG-ReportStyle" {
            n166 = case shown="\"Metric\", Default" w532 {
              tunnel: [w542 w552] -> w535
              tunnel: [w541 w551] -> w534
              tunnel: [w540 w550] -> w533
              tunnel: w531 -> [w539 w549]
              frame "Metric", Default {
                n167 = case shown="False" w539 {
                  tunnel: ["h= %.3f" ("format string") "h= %.0{m}f" ("format string")] -> w542
                  tunnel: ["U(h)= %0.2{m/s}f" ("format string") "U(h)= %0.2{m/s}f" ("format string")] -> w541
                  tunnel: ["λ= %0.3f" ("format string") "λ= %0.0{m}f" ("format string")] -> w540
                  frame False {
                  }
                  frame True {
                  }
                }
              }
              frame "English" {
                n168 = case shown="False" w549 {
                  tunnel: ["h= %.0{ft}f" ("format string") "h= %.1{in}f" ("format string")] -> w552
                  tunnel: ["U(h)= %0.1{ft/s}f" ("format string") "U(h)= %0.1{ft/s}f" ("format string")] -> w551
                  tunnel: ["λ= %0.0{ft}f" ("format string") "λ= %0.1{in}f" ("format string")] -> w550
                  frame True {
                  }
                  frame False {
                  }
                }
              }
            }
          }
        }
        n169 = local read "lambda(h)"() -> (w503:dbl)
        n170 = local read "U(h)"() -> (w500:dbl[unit])
        n171 = global read "Results_plotter_Global.vi" "Scale"() -> (w484:u16)
        n172 = node(w503) -> (w480:dbl[unit])
        n173 = Multiply(x=w484, y="h") -> (x*y=w486:dbl[unit])
        n174 = Multiply(x=w484, y=w480) -> (x*y=w485:dbl[unit])
        n175 = Format Into String(format string=w493, w486) -> (resulting string=w492:string)  [unwired: 2 in, 1 out]
        n176 = Format Into String(format string=w491, w500) -> (resulting string=w490:string)  [unwired: 2 in, 1 out]
        n177 = Format Into String(format string=w489, w485) -> (resulting string=w488:string)  [unwired: 2 in, 1 out]
        n178 = call "SetSizeAndOriginForMultiplot.vi"("VerticalPosition"=w509, "Height"=w497, "LateralPosition"=w509, "Width"=w508, "ClearLabels?"=TRUE, "PlotLocationDescription"="Bottom plot", "gnuplotIn"=w510) -> ("gnuplotOut"=w505:string)  [unwired: 4 in]
        n179 = Build Array(w492, w490, w488) -> (w499:string[])
        n180 = call "setLabel.vi"("\"At\" location"=T5 {"XcoordSys"="graph", "YcoordSys"="graph", "Xvalue"=0.98, "Yvalue"=0.85} ("\"At\" location"), "Justify"="right", "multilineLabel"=w499, "String in"=w505) -> ("String out"=w504:string)  [unwired: 6 in, 1 out]
        n181 = control-ref of="Spectrum"() -> (w518:refnum<vi>)
        n182 = call "getAxisBounds.vi"("Active Y Scale"=w515, "Active X Scale"=w515, "XYGraph in"=w518) -> ("Ybounds"=w516:T10, "Xbounds"=w517:T10)  [unwired: 5 in, 2 out]
        n183 = call "AssembleBLMultiplotScript-Spectra.vi"("gnuplotIn"=w504, "Title"=w496, "SpectrumFilename"=w513, "f.E(f) Bounds"=w516, "f Bounds"=w517) -> ("gnuplotOut"=w514:string)  [unwired: 10 in]
      }
      frame "Write gnuplot file" {
        w573 = FALSE  # append to file? (new file:F)
        w574 = FALSE  # advisory dialog? (display:T)
        n184 = call "chainCommands.vi"("Command"="unset multiplot\t", "Comments"="Close out multiplot", "StringIn"=w561) -> ("StringOut"=w560:string)  [unwired: 8 in]
        n185 = Build Path(base path=w566, name or relative path="gnuplot_script.txt") -> (appended path=w575:path)
        n186 = call "Write_Characters_To_File.vi"("file path (dialog if empty)"=w575, "advisory dialog? (display:T)"=w574, "character string"=w560, "append to file? (new file:F)"=w573) -> ()  [unwired: 1 in, 4 out]
      }
      frame "Execute shell script" {
        n187 = disable-structure shown="Enabled" {
          disable-tunnel: [w592 w599] -> w579
          frame Disabled {
            n188 = local read "Final Title"() -> (w594:string)
            n189 = Search and Replace String(replace all?=TRUE ("replace all? (F)"), input string=w594, search string=" ", replace string="\\ " ("replace string (\"\")")) -> (result string=w593:string)  [unwired: 4 in, 3 out]
            n190 = call <vilib>:"Is Name Multiplatform.vi"("filename must be valid on all platforms (F)"=TRUE ("name must work for all platforms (F)"), "filename"=w593) -> ("suggested filename"=w592:string)  [unwired: 5 in, 4 out]
          }
          frame Enabled {
            n191 = local read "FileName"() -> (w599:string)
          }
        }
        n192 = local read "OutputType"() -> (w580:enum16{"PDF", "PNG-ReportStyle"})
        n193 = Build Path(base path=w578, name or relative path=w579) -> (appended path=w577:path)
        n194 = call "Run_Gnuplot_Script.vi"("OutputType"=w580, "logfileName"=w586, "targetFile"=w577) -> ()
      }
      frame "Has pdf been generated?" {
        n195 = Select(t="Open Standard output file" ("f"), s="OpenLogfile?", f="UI-Monitor" ("t")) -> (s? t:f=w608:string)
        n196 = Select(t="Show Re-Run Gnuplot?", s="Show Script Editor?", f=w608) -> (s? t:f=w611:string)
        n197 = local read "autoprint"() -> (w601:bool)
        n198 = Not(x=w601) -> (.not. x?=w602:bool)
      }
      frame "Show Re-Run Gnuplot?" {
        n199 = local read "OutputType"() -> (w618:enum16{"PDF", "PNG-ReportStyle"})
        n200 = call "Re_run_Gnuplot.vi"("Plot folder (dialog if empty)"=w623, "OutputType"=w618) -> ()  [unwired: 3 out]
      }
      frame "Open Standard output file" {
        n201 = Format Into String(format string="open \"%s\"", w637) -> (resulting string=w636:string)  [unwired: 2 in, 1 out]
        n202 = call <vilib>:"System Exec.vi"("working directory"=w633, "command line"=w636) -> ()  [unwired: 4 in, 6 out]
      }
    }
    "case" <- w30
    "gnuplotScript" <- w27
    "outputPath" <- w15
    n203 = Compound Arithmetic op=AND(w10, invert "Stop Button") -> (w9:bool)
  }
  n204 = local write "Stop Button"(w2) -> ()
  "Saved Automatically?" <- FALSE
